vi "test_ThreeSessThreePinTwoInstrTwoSiteReservation_CallGetConnectionFromPinForOneDcPowerPinAllSites_ReturnsMulitpleConnectionsError.vi"(8 "error in":errorcluster) -> (0 "error out":errorcluster, 2 "result":string, 3 "pass":bool)   [LabVIEW 2020, in "MeasurementServerTests.lvlib"]
uses:
  MeasurementServerTests.lvlib
  Runtime/MeasurementLink Session Management V1/Session Reservation/Connection.ctl
  Runtime/MeasurementLink Session Management V1/Session Reservation/Session Reservation.lvclass
  Runtime/MeasurementLink Session Management V1/Session Reservation/Connection with Session.ctl
  Runtime/MeasurementLink Measurement Server/Helpers/Error Strings Global Internal.vi
  933abbf5-676f-4ffb-8d63-f5b1913fa17d.vi
  Runtime/MeasurementLink niDCPower/Session Factory/Session Factory.lvclass
  Runtime/MeasurementLink Session Management V1/Session Reservation/Pin Type.ctl
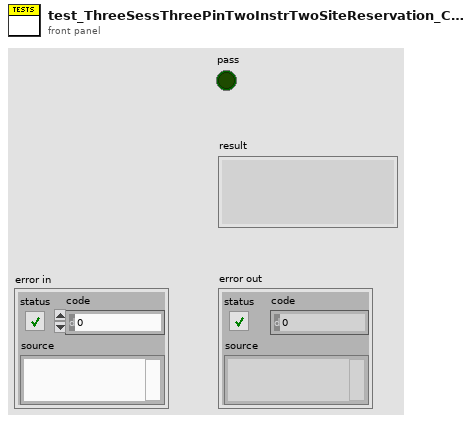
[diagram p1: front panel]
types:
  T1 = typedef "MeasurementLink Session Management V1.lvlib/Session Reservation.lvclass/Pin Type.ctl" = enum16{"DUT and System Pins", "System Pins"}
  T2 = typedef "MeasurementLink Session Management V1.lvlib/Session Reservation.lvclass/Connection with Session.ctl" = cluster{"connection":T3, "session":variant}
  T3 = typedef "MeasurementLink Session Management V1.lvlib/Session Reservation.lvclass/Connection.ctl" = cluster{"pin or relay name":string, "site":i32, "instrument type id":string, "channel":string}
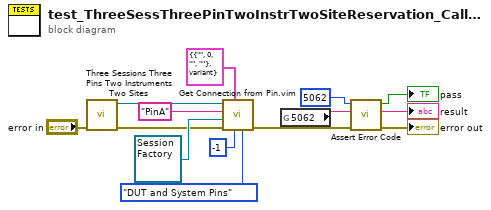
[diagram p0: block diagram]
diagram:
  n1 = call "Three Sessions Three Pins Two Instruments Two Sites.vi"("error in"="error in") -> ("error out"=w1:errorcluster, "session reservation out"=w2:refnum<class "Session Reservation.lvclass">)  [unwired: 8 in, 1 out]
  n2 = call "Get Connection from Pin.vim"("pin type"=Pin_Type."DUT and System Pins", "site"=-1, "connection type"=T2 {"connection"={"pin or relay name"="", "site"=0, "instrument type id"="", "channel"=""}, "session"=variant} ("connection"), "error in"=w1, "session factory"=refnum<class "Session Factory.lvclass"> refnum ("MeasurementLink niDCPower.lvlib:Instrument.lvclass"), "pin or relay name"="PinA", "session reservation in"=w2) -> ("error out"=w9:errorcluster)  [unwired: 2 in, 2 out]
  n3 = global read "Error Strings Global Internal.vi" "5062"() -> (w10:string)
  n4 = call "Assert Error Code.vi"("error in"=w9, "expected error description"=w10, "expected error code"=5062) -> ("error out"=→"error out":errorcluster, "details"=→"result":string, "error code match?"=→"pass":bool)  [unwired: 6 in]
